vi "Untitled 3.vi"() -> ()   [LabVIEW 2020]
uses:
  Labview Library/Libraries/Basic Experiment/Scan Settings.ctl
  Axis Enum.ctl
  Labview Library/Libraries/Save Module/Libraries/Save Module/Save Module.lvlib
  Labview Library/Libraries/Basic Experiment/Basic Experiment.lvlib
panel:
  in  "file path":path=path "G:/Default/Save/dd.tdms"
  in  "Scan parameter":T1={"Horizontal axis"=enum."x", "Vertical axis"=enum."y", "vertical num"=100, "vertical end"=50.0, "vertical start"=40.0, "horizontal num"=100, "horizontal end"=25.0, "horizontal start"=15.0}
  in  "Intensity Graph":dbl[][](graph)=array101x101[10201 elements]
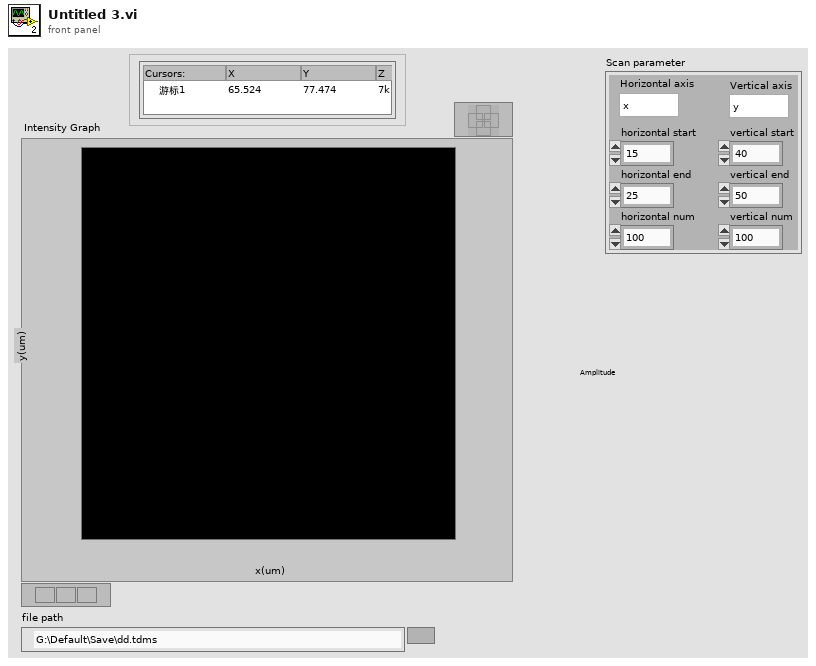
[diagram p1: front panel]
types:
  T1 = typedef "Basic Experiment.lvlib/Scan Settings.ctl" = cluster{"Horizontal axis":T2, "Vertical axis":T2, "vertical num":u32, "vertical end":dbl, "vertical start":dbl, "horizontal num":u32, "horizontal end":dbl, "horizontal start":dbl}
  T2 = typedef "Axis Enum.ctl" = enum16{"x", "y", "z"}
  T3 = enum16{"open", "open or create", "create or replace", "create", "open (read-only)"}
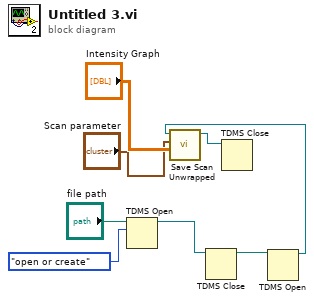
[diagram p0: block diagram]
diagram:
  n1 = TDMS Open(10:T3."open or create" ("operation (0:open)"), 11:"file path") -> (3:w3:refnum<k34>)  [unwired: 5 in, 1 out]
  n2 = TDMS Close(11:w3) -> (3:w2:path)  [unwired: 1 in, 1 out]
  n3 = TDMS Open(11:w2) -> (3:w1:refnum<k34>)  [unwired: 6 in, 1 out]
  n4 = call "Save Scan Unwrapped.vi"("Intensity Graph"="Intensity Graph", "Scan parameter"="Scan parameter", "tdms file"=w1) -> ("tdms file out"=w6:refnum<k34>)  [unwired: 8 in]
  n5 = TDMS Close(11:w6) -> ()  [unwired: 1 in, 2 out]
